vi "FPGATorque.vi"(2 "Calib Pt 1 (ft-lbf)":sgl, 3 "Calib Pt 1 (amps)":sgl, 4 "Calib Pt 0 (ft-lbf)":sgl, 5 "Calib Pt 0 (amps)":sgl) -> (0 "Top Drive Torque":sgl, 1 "Mod3-9203/AI0":sgl)   [LabVIEW 2019]
uses:
  <vilib>/rvi/eio/common/nirviEmuTemplateMethod_errors.vi
  <vilib>/eio/EIONode/EIONode.xnode
panel:
  # "READ Torque Sensor"
  # "StraightPoint Custom Load Pin"
  # "(Amps)"
  # "Torque (ft-lbf)"
  # "Calibration Data"
  # "Specification Data"
  # "Spec Pt 0 (0 lbf) = 4 mA"
  # "Spec Pt 1 (1240 lbf) = 20 mA"
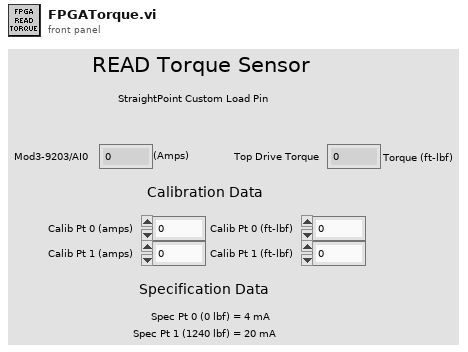
[diagram p1: front panel]
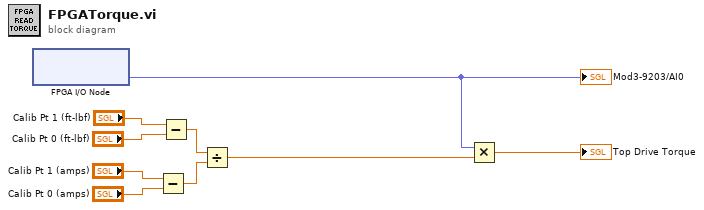
[diagram p0: block diagram]
diagram:
  n1 = xnode "FPGA I/O Node"() -> ("Mod3/AI0"=w3:fxp<+/-,21,-4>)  [unwired: 1 in, 1 out]
  "Mod3-9203/AI0" <- w3
  n2 = Subtract(x="Calib Pt 1 (amps)", y="Calib Pt 0 (amps)") -> (x-y=w6:sgl)
  n3 = Subtract(x="Calib Pt 1 (ft-lbf)", y="Calib Pt 0 (ft-lbf)") -> (x-y=w8:sgl)
  n4 = Divide(x=w8, y=w6) -> (x/y=w2:sgl)
  n5 = Multiply(x=w3, y=w2) -> (x*y=→"Top Drive Torque":sgl)
